vi "Select Physical Channels.vi"(11 "Physical Channels In":bool[](array[boolean])) -> (2 "Cancelled?":bool, 3 "Physical Channels Out":bool[](array[boolean]))   [LabVIEW 2020, in "Waveform Analog Output System Explorer.lvlib"]
doc: "When called, launches a dialogue to select AO channels to be added to the system definition"
uses:
  Waveform Analog Output System Explorer.lvlib
panel:
  in  "Cancel":bool
  in  "Accept":bool
  in  "Physical Channels":T1
  # "Please Select the Channels to Use"
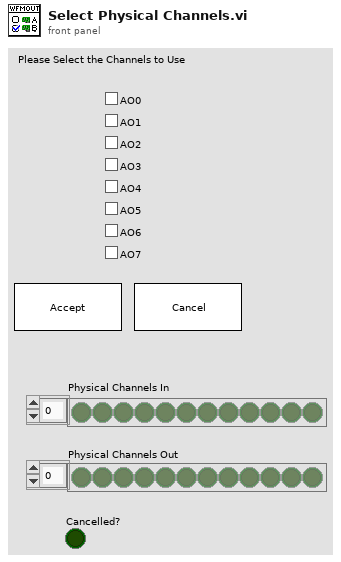
[diagram p1: front panel]
types:
  T1 = cluster{"AO0":bool, "AO1":bool, "AO2":bool, "AO3":bool, "AO4":bool, "AO5":bool, "AO6":bool, "AO7":bool}
  T2 = cluster{"Physical Channels In[0]":bool, "Physical Channels In[1]":bool, "Physical Channels In[2]":bool, "Physical Channels In[3]":bool, "Physical Channels In[4]":bool, "Physical Channels In[5]":bool, "Physical Channels In[6]":bool, "Physical Channels In[7]":bool}
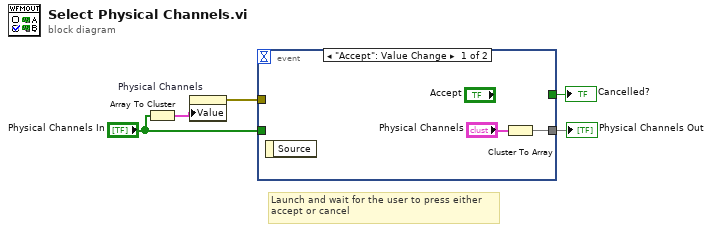
[diagram p0: block diagram]
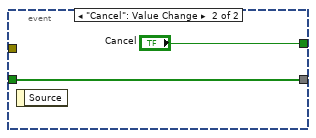
[diagram p2: hidden frame]
diagram:
  # "Launch and wait for the user to press either\naccept or cancel"
  n1 = Array To Cluster(array="Physical Channels In") -> (cluster=w3:T2)
  n2 = property on="Physical Channels" class="Clust (strict)"("Value"=w3) -> (error out=w2:errorcluster)  [unwired: 2 in, 1 out]
  n3 = event shown="[0] \"Accept\": Value Change" {
    selector: _ -> [_ _]
    dyn-events: _ -> [_ _]
    timeout: _ -> [_ _]
    tunnel: [w6 w9] -> w5
    tunnel: "Physical Channels In" -> [_ w9]
    tunnel: w2 -> [_ _]
    tunnel: [_ "Cancel"] -> w1
    event "Accept": Value Change {
      n4 = event-data() -> ()  [unwired: 1 in, 1 out]
      n5 = Cluster To Array(cluster="Physical Channels") -> (array=w6:bool[])
    }
    event "Cancel": Value Change {
      n6 = event-data() -> ()  [unwired: 1 in, 1 out]
    }
  }
  "Physical Channels Out" <- w5
  "Cancelled?" <- w1
